vi "Ensure Default Font.vi"(8 "error in":errorcluster, 11 "SpreadsheetDoc in":refnum<k24>) -> (0 "error out":errorcluster, 3 "SpreadsheetDoc out":refnum<k24>)   [LabVIEW 2019, in "Open Xml.lvlib"]
uses:
  Open Xml.lvlib
  D:/git/Open-Xml-LabVIEW/Source/DocumentFormat.OpenXml.dll
  DocumentFormat.OpenXml.dll
  D:/git/Open-Xml-LabVIEW/Source/DocumentFormat.OpenXml.Framework.dll
  DocumentFormat.OpenXml.Framework.dll
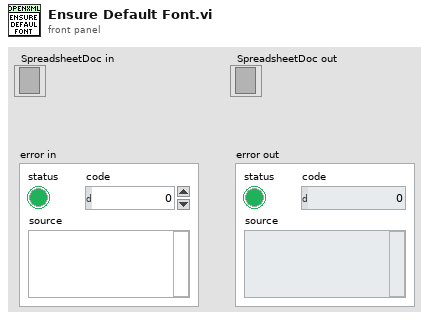
[diagram p1: front panel]
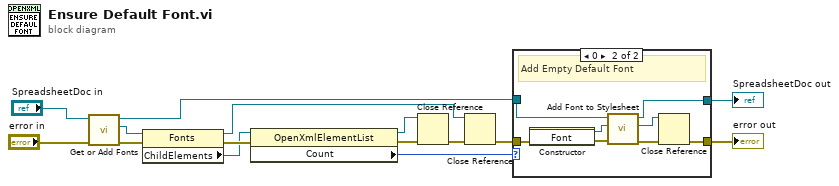
[diagram p0: block diagram]
diagram:
  n1 = call "Get or Add Fonts.vi"("error in"="error in", "SpreadsheetDoc in"="SpreadsheetDoc in") -> ("error out"=w11:errorcluster, "Fonts"=w10:refnum<k24>, "SpreadsheetDoc out"=w7:refnum<k24>)  [unwired: 7 in]
  n2 = property class="Fonts"(reference=w10, error in=w11) -> (reference out=w2:refnum<k24>, error out=w9:errorcluster, "ChildElements"=w4:refnum<k24>)
  n3 = property class="OpenXmlElementList"(reference=w4, error in=w9) -> (reference out=w1:refnum<k24>, error out=w6:errorcluster, "Count"=w8:i32)
  n4 = Close Reference(reference=w1, error in (no error)=w6) -> (error out=w5:errorcluster)
  n5 = Close Reference(reference=w2, error in (no error)=w5) -> (error out=w3:errorcluster)
  n6 = case shown="0" w8 {
    tunnel: w7 -> [w16 w25]
    tunnel: w3 -> [w17 w24]
    tunnel: [w17 w19] -> w14
    tunnel: [w16 w21] -> w15
    frame Default {
      # "Default"
    }
    frame 0 {
      # "Add Empty Default Font"
      n7 = constructor class="Font"(error in=w24) -> (reference out=w22:refnum<k24>, error out=w23:errorcluster)  [unwired: 2 in, 1 out]
      n8 = call "Add Font to Stylesheet.vi"("error in"=w23, "Font in"=w22, "SpreadsheetDoc in"=w25) -> ("error out"=w20:errorcluster, "Font out"=w18:refnum<k24>, "SpreadsheetDoc out"=w21:refnum<k24>)  [unwired: 5 in, 1 out]
      n9 = Close Reference(reference=w18, error in (no error)=w20) -> (error out=w19:errorcluster)
    }
  }
  "SpreadsheetDoc out" <- w15
  "error out" <- w14
